vi "产品SN消息解析.vi"(8 "SN":string="SN111111", 9 "body":string, 11 "消息框":refnum<vi>) -> ()   [LabVIEW 2015]
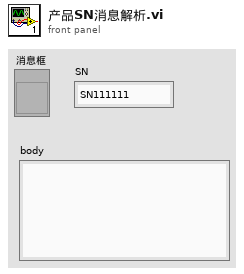
[diagram p1: front panel]
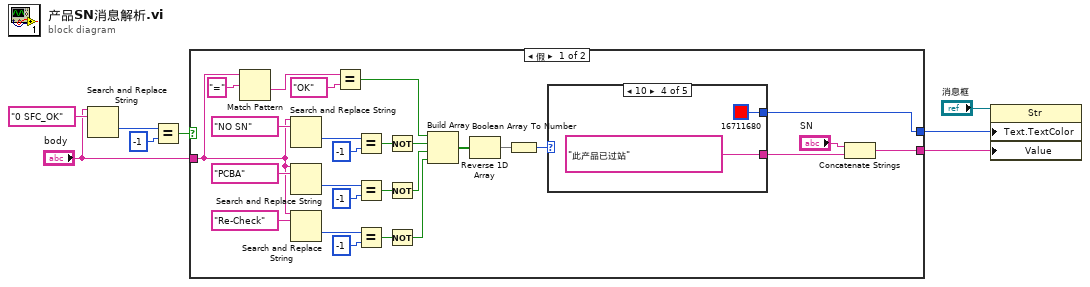
[diagram p0: block diagram]
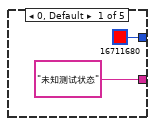
[diagram p2: hidden frame]
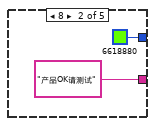
[diagram p3: hidden frame]
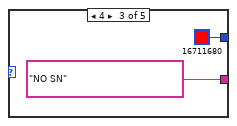
[diagram p4: hidden frame]
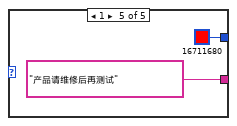
[diagram p5: hidden frame]
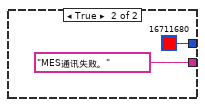
[diagram p6: hidden frame]
diagram:
  n1 = Search and Replace String(input string="body", search string="0 SFC_OK") -> (offset past replacement=w7:i32)  [unwired: 6 in, 3 out]
  n2 = Equal?(x=w7, y=-1) -> (x = y?=w4:bool)
  n3 = case shown="假" w4 {
    tunnel: [w12 "MES通讯失败。"] -> w3
    tunnel: [w10 u32 16711680] -> w2
    tunnel: "body" -> [w29 _]
    frame False {
      n4 = Match Pattern(string=w29, regular expression="=" ("正则表达式")) -> (after substring=w35:string)  [unwired: 1 in, 3 out]
      n5 = Search and Replace String(input string=w29, search string="NO SN") -> (offset past replacement=w27:i32)  [unwired: 6 in, 3 out]
      n6 = Search and Replace String(input string=w29, search string="PCBA") -> (offset past replacement=w25:i32)  [unwired: 6 in, 3 out]
      n7 = Search and Replace String(input string=w29, search string="Re-Check") -> (offset past replacement=w24:i32)  [unwired: 6 in, 3 out]
      n8 = Equal?(x=w35, y="OK") -> (x = y?=w22:bool)
      n9 = Equal?(x=w27, y=-1) -> (x = y?=w21:bool)
      n10 = Equal?(x=w25, y=-1) -> (x = y?=w20:bool)
      n11 = Equal?(x=w24, y=-1) -> (x = y?=w19:bool)
      n12 = Not(x=w21) -> (.not. x?=w18:bool)
      n13 = Not(x=w20) -> (.not. x?=w17:bool)
      n14 = Not(x=w19) -> (.not. x?=w16:bool)
      n15 = Build Array(w22, w18, w17, w16) -> (w15:bool[])
      n16 = Reverse 1D Array(array=w15) -> (reversed array=w9:bool[])
      n17 = Boolean Array To Number(Boolean array=w9) -> (number=w14:u32)
      n18 = case shown="10" w14 {
        tunnel: ["未知测试状态" "产品OK请测试" "NO SN" "此产品已过站" "产品请维修后再测试"] -> w11
        tunnel: [u32 16711680 u32 6618880 u32 16711680 u32 16711680 u32 16711680] -> w10
        frame 0, Default {
        }
        frame 8 {
        }
        frame 4 {
        }
        frame 2 {
        }
        frame 1 {
        }
      }
      n19 = Concatenate Strings("SN", w11) -> (w12:string)
    }
    frame True {
    }
  }
  n20 = property class="Str"(reference="消息框", "Text.TextColor"=w2, "Value"=w3) -> ()  [unwired: 1 in, 2 out]
